vi "Set Output Node Parameters.vi"(4 "Apply parameters":bool=TRUE, 5 "Enable":i32=1, 6 "Use Enable":bool, 7 "Node parameters":T1, 8 "error in (no error)":errorcluster, 9 "node":i32, 10 "idxChannel":i32, 11 "hdwf":i32) -> (0 "error out":errorcluster, 1 "x .and. y?":i32)   [LabVIEW 2024, in "AD2 DLL.lvlib"]
uses:
  AD2 DLL.lvlib
  Node Parameters.ctl
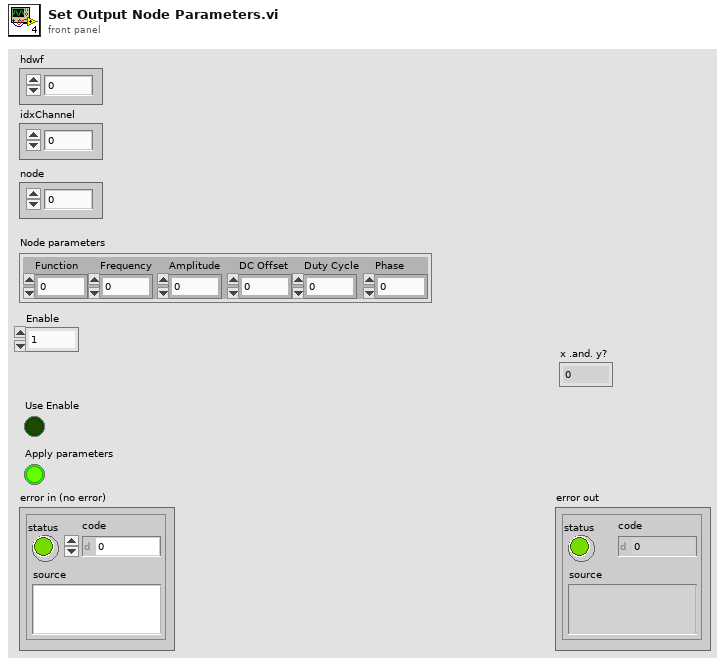
[diagram p1: front panel]
types:
  T1 = typedef "AD2 DLL.lvlib/Node Parameters.ctl" = cluster{"Function":u8, "Frequency":dbl, "Amplitude":dbl, "DC Offset":dbl, "Duty Cycle":dbl, "Phase":dbl}
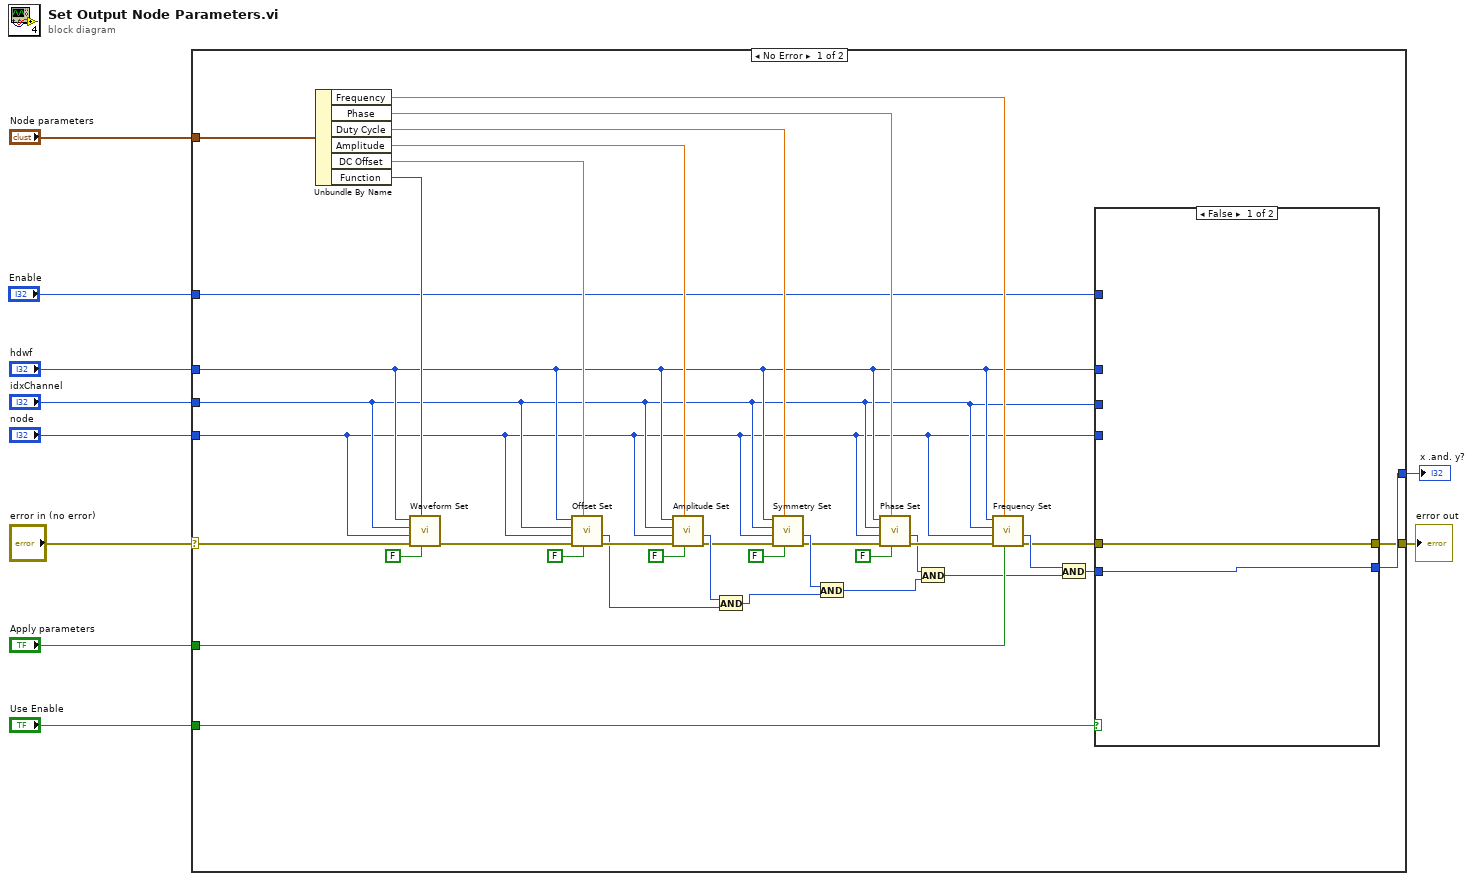
[diagram p0: block diagram]
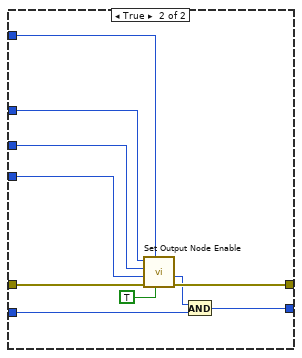
[diagram p2: hidden frame]
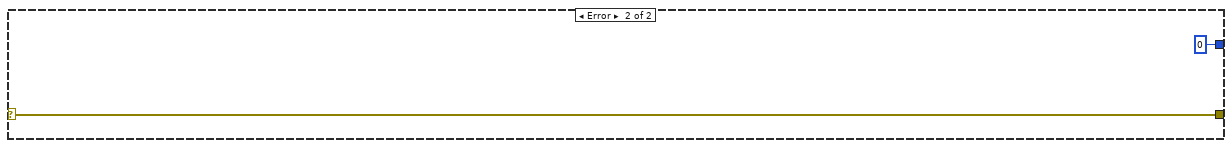
[diagram p3: hidden frame]
diagram:
  n1 = case shown="No Error" "error in (no error)" {
    selector: "error in (no error)" -> [w11 w60]
    tunnel: "Apply parameters" -> [w43 _]
    tunnel: "Node parameters" -> [w37 _]
    tunnel: [w19 0] -> w8
    tunnel: "Use Enable" -> [w18 _]
    tunnel: [w16 w60] -> w6
    tunnel: "hdwf" -> [w15 _]
    tunnel: "idxChannel" -> [w14 _]
    tunnel: "node" -> [w13 _]
    tunnel: "Enable" -> [w12 _]
    frame No Error {
      n2 = Unbundle By Name(w37) -> ("Frequency"=w36:dbl, "Phase"=w25:dbl, "Duty Cycle"=w28:dbl, "Amplitude"=w35:dbl, "DC Offset"=w34:dbl, "Function"=w33:u8)
      n3 = call "Waveform Set.vi"("Update"=FALSE, "Function"=w33, "error in (no error)"=w11, "node"=w13, "idxChannel"=w14, "hdwf"=w15) -> ("error out"=w39:errorcluster)  [unwired: 4 in, 1 out]
      n4 = call "Offset Set.vi"("Update"=FALSE, "Offset"=w34, "error in (no error)"=w39, "node"=w13, "idxChannel"=w14, "hdwf"=w15) -> ("error out"=w46:errorcluster, "func_out"=w42:i32)  [unwired: 3 in, 1 out]
      n5 = call "Amplitude Set.vi"("Update"=FALSE, "Amplitude"=w35, "error in (no error)"=w46, "node"=w13, "idxChannel"=w14, "hdwf"=w15) -> ("error out"=w32:errorcluster, "func_out"=w41:i32)  [unwired: 3 in, 1 out]
      n6 = And(x=w41, y=w42) -> (x .and. y?=w30:i32)
      n7 = call "Symmetry Set.vi"("Update"=FALSE, "Duty Cycle"=w28, "error in (no error)"=w32, "node"=w13, "idxChannel"=w14, "hdwf"=w15) -> ("error out"=w27:errorcluster, "func_out"=w29:i32)  [unwired: 3 in, 1 out]
      n8 = And(x=w29, y=w30) -> (x .and. y?=w24:i32)
      n9 = call "Phase Set.vi"("Update"=FALSE, "Phase Cycle"=w25, "error in (no error)"=w27, "node"=w13, "idxChannel"=w14, "hdwf"=w15) -> ("error out"=w26:errorcluster, "func_out"=w23:i32)  [unwired: 3 in, 1 out]
      n10 = And(x=w23, y=w24) -> (x .and. y?=w22:i32)
      n11 = call "Frequency Set.vi"("Update"=w43, "Frequency"=w36, "error in (no error)"=w26, "node"=w13, "idxChannel"=w14, "hdwf"=w15) -> ("error out"=w17:errorcluster, "func_out"=w40:i32)  [unwired: 3 in, 1 out]
      n12 = And(x=w40, y=w22) -> (x .and. y?=w20:i32)
      n13 = case shown="False" w18 {
        tunnel: w20 -> [w47 w53]
        tunnel: [w47 w51] -> w19
        tunnel: w17 -> [w48 w58]
        tunnel: [w48 w57] -> w16
        tunnel: w15 -> [_ w56]
        tunnel: w14 -> [_ w55]
        tunnel: w13 -> [_ w54]
        tunnel: w12 -> [_ w50]
        frame False {
        }
        frame True {
          n14 = call "Set Output Node Enable.vi"("Update"=TRUE, "Enable"=w50, "error in (no error)"=w58, "node"=w54, "idxChannel"=w55, "hdwf"=w56) -> ("error out"=w57:errorcluster, "func_out"=w52:i32)  [unwired: 4 in]
          n15 = And(x=w52, y=w53) -> (x .and. y?=w51:i32)
        }
      }
    }
    frame Error {
    }
  }
  "error out" <- w6
  "x .and. y?" <- w8
